vi "xml generate for SFP+_VNA_Full - 副本.vi"(0 "input_array_SDD11_Max":string[](array[string]), 2 "路径":path=path "D:/wmgxml.xml", 3 "input_str_label":string, 4 "input_str_CustomerPN":string, 5 "input_array_SCC11_Max":string[](array[string]), 6 "FilePath":string, 7 "input_array_ILD_Max":string[](array[string]), 8 "FileVer":string, 9 "input_array_TDD11":string[](array[string]), 11 "input_array_TDD22":string[](array[string]), 13 "input_array_time":string[](array[string]), 14 "input_array_impSpec":string[](array[string])) -> ()   [LabVIEW 2011]
panel:
  in  "input_path_dataSource":path
  out "TDD":string
  out "NEXT":string
  out "SCC11":string
  out "SCD21-SDD21":string
  out "ILD":string
  out "SDD11":string
  out "SDD21":string
  in  "RawTXTPath":path
  in  "input_test_results":bool[](array[boolean])
  out "midVar_time":string[](array[string])
  in  "midVar_state":string
  in  "input_str_product":string
  out "midVar_Content":string
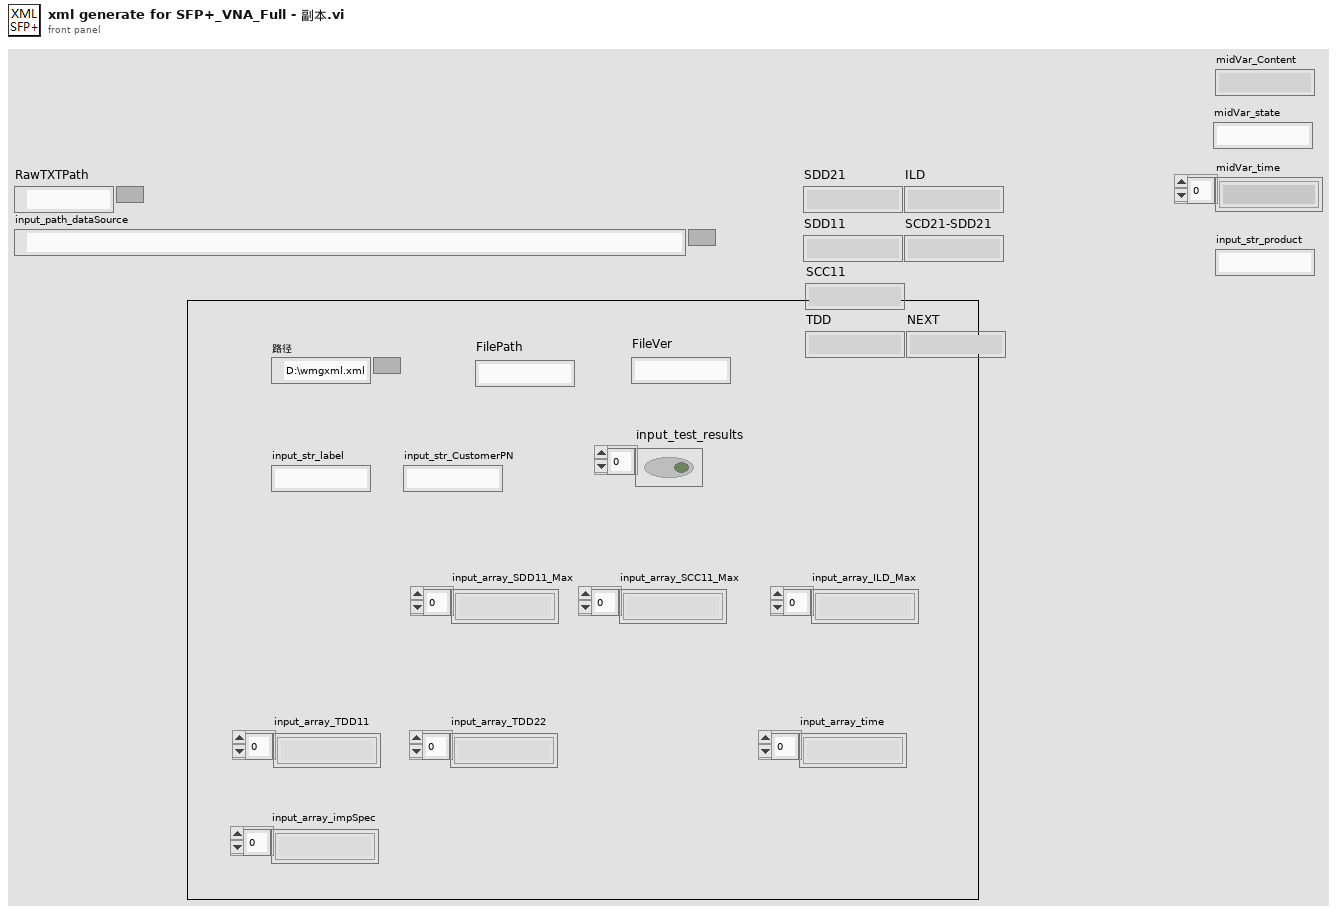
[diagram p1: front panel]
types:
  T1 = enum16{"open", "replace", "create", "open or create", "replace or create", "replace or create with confirmation"}
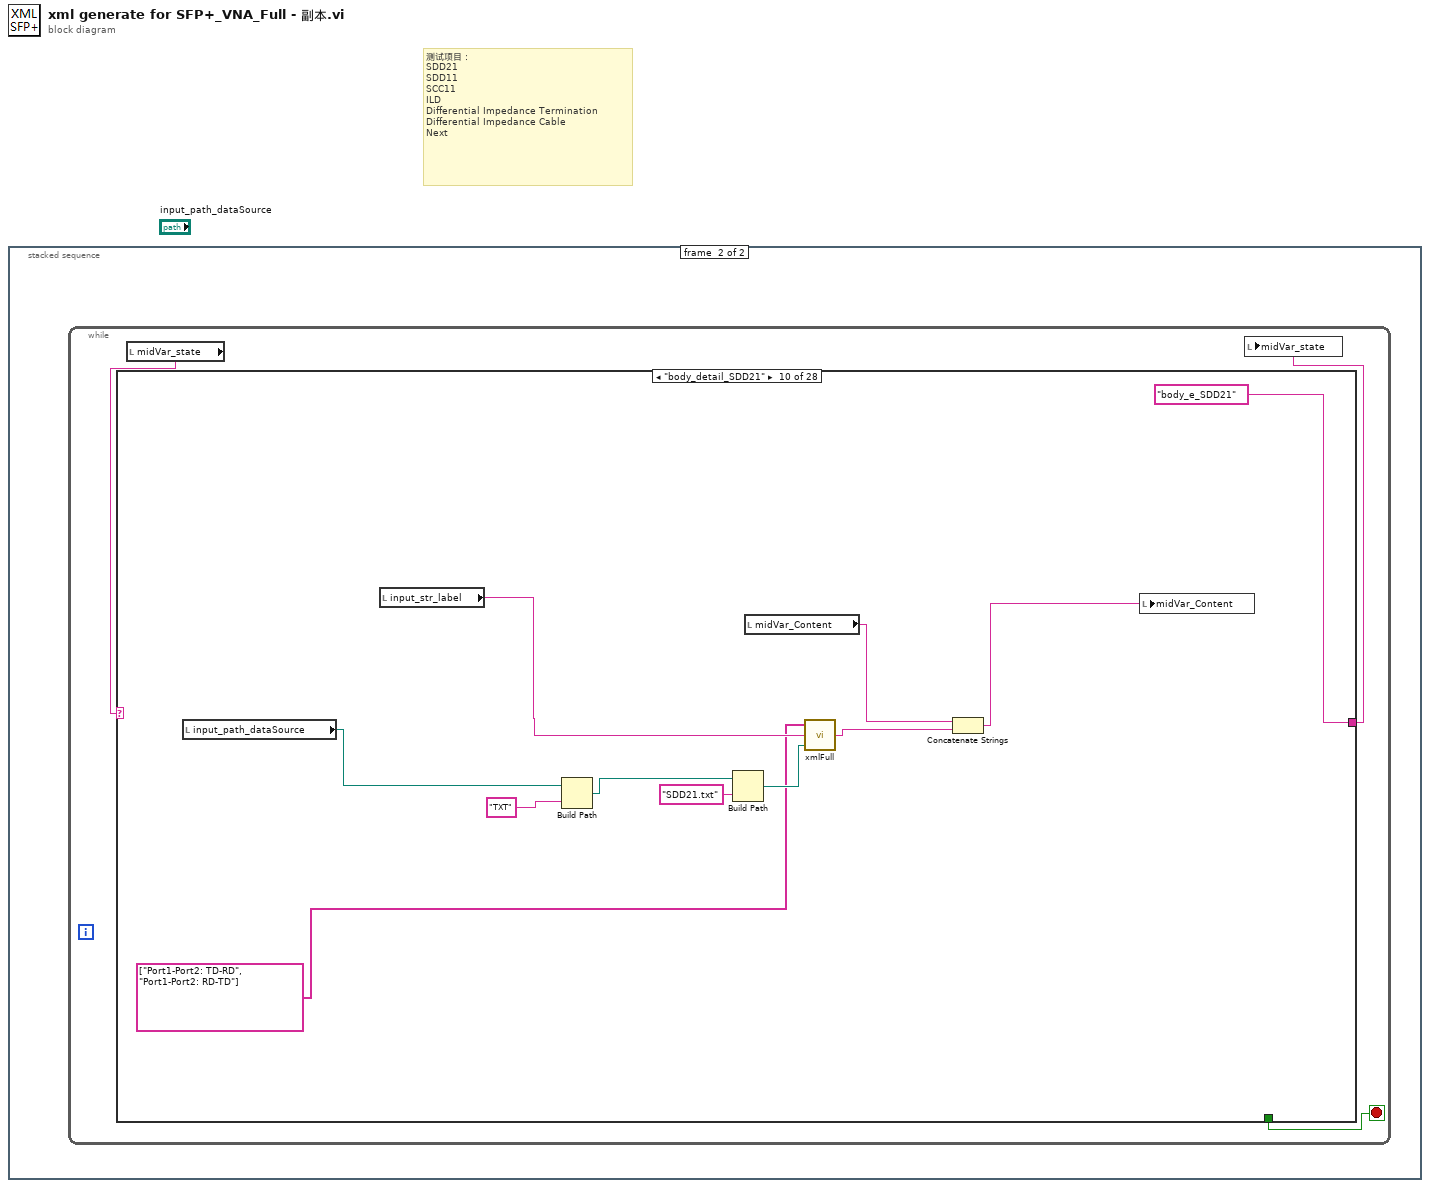
[diagram p0: block diagram]
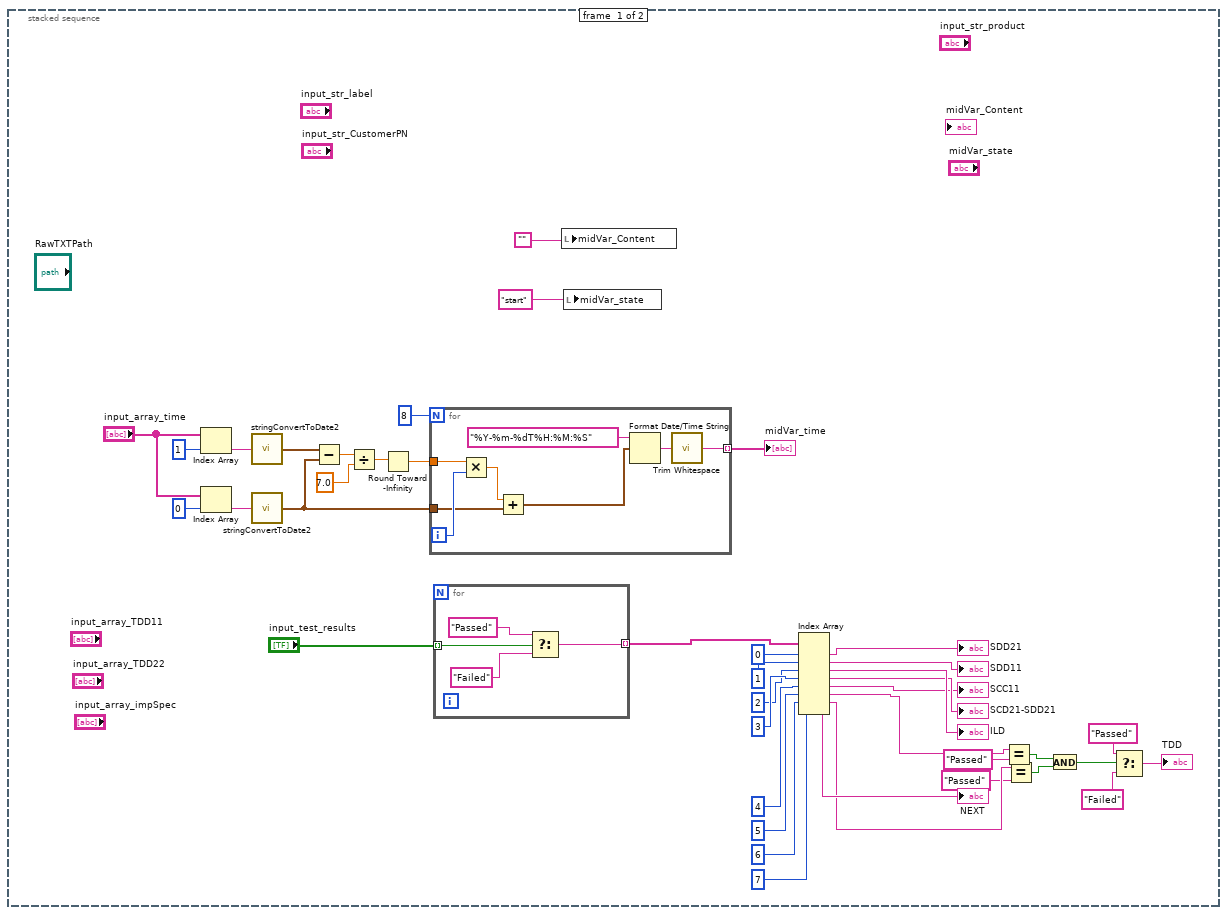
[diagram p2: hidden frame]
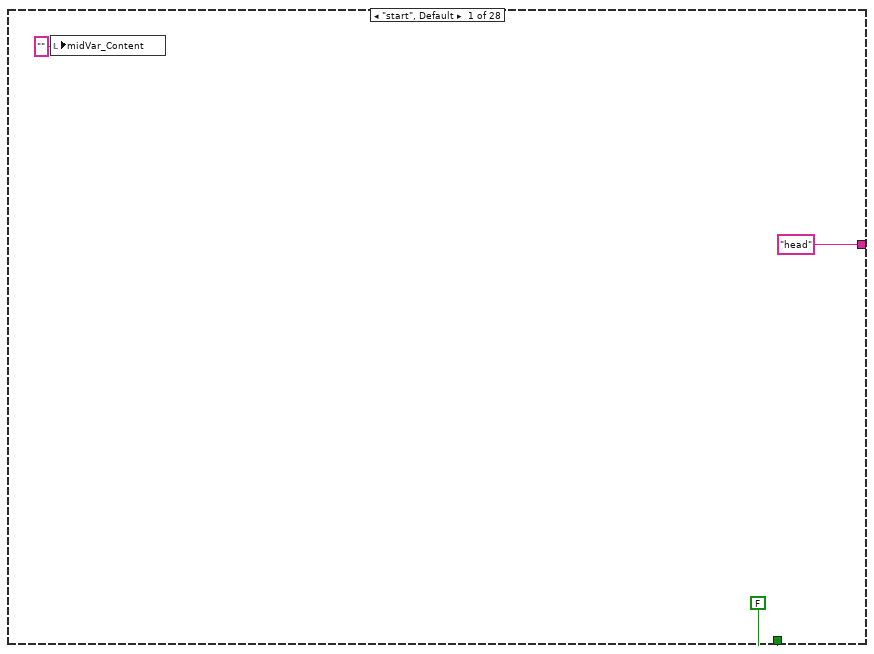
[diagram p3: hidden frame]
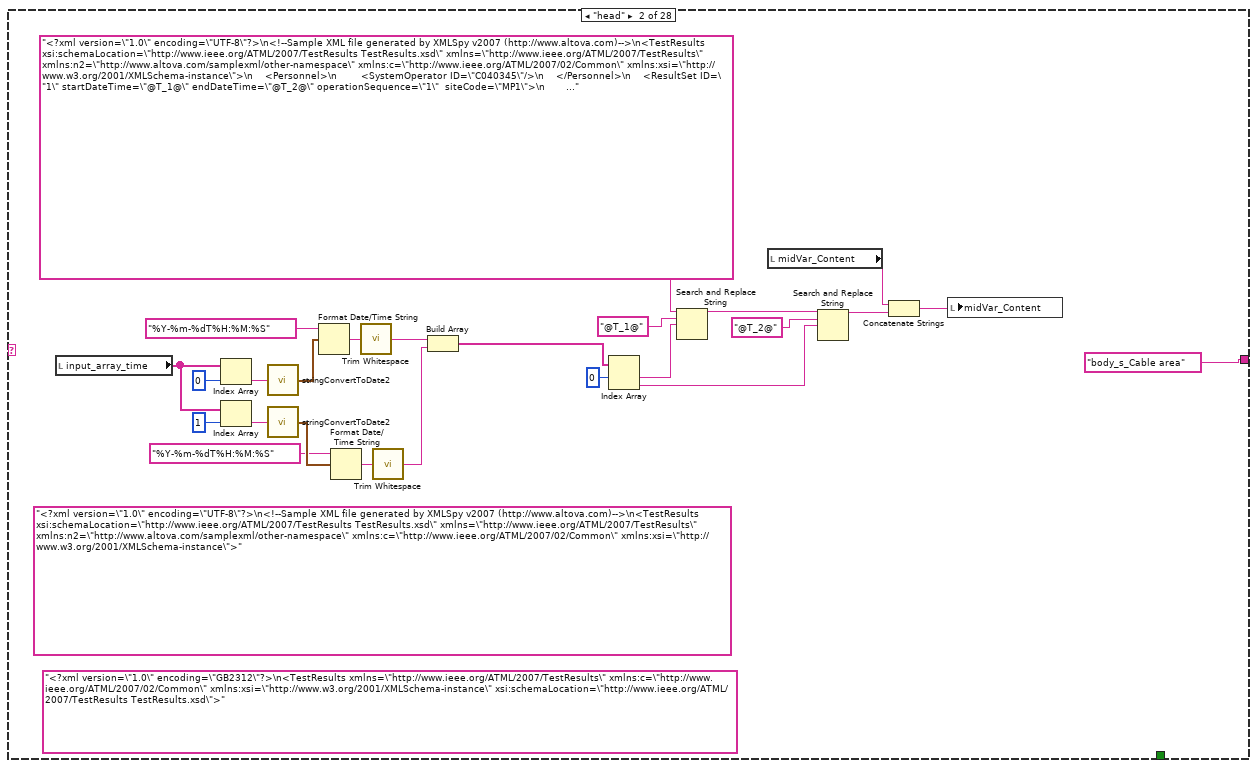
[diagram p4: hidden frame]
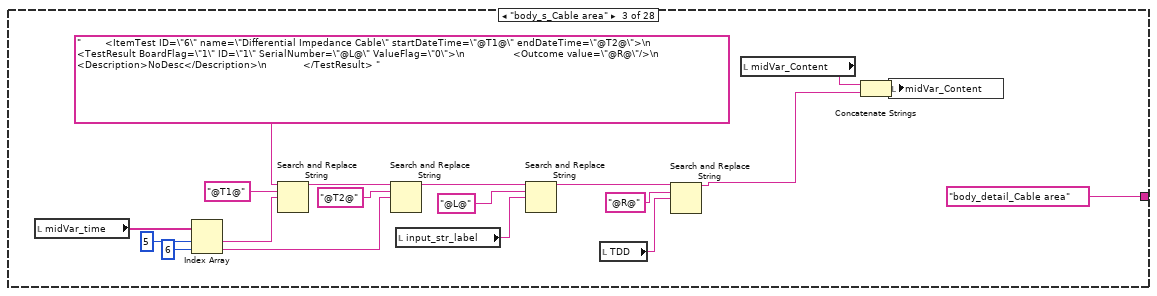
[diagram p5: hidden frame]
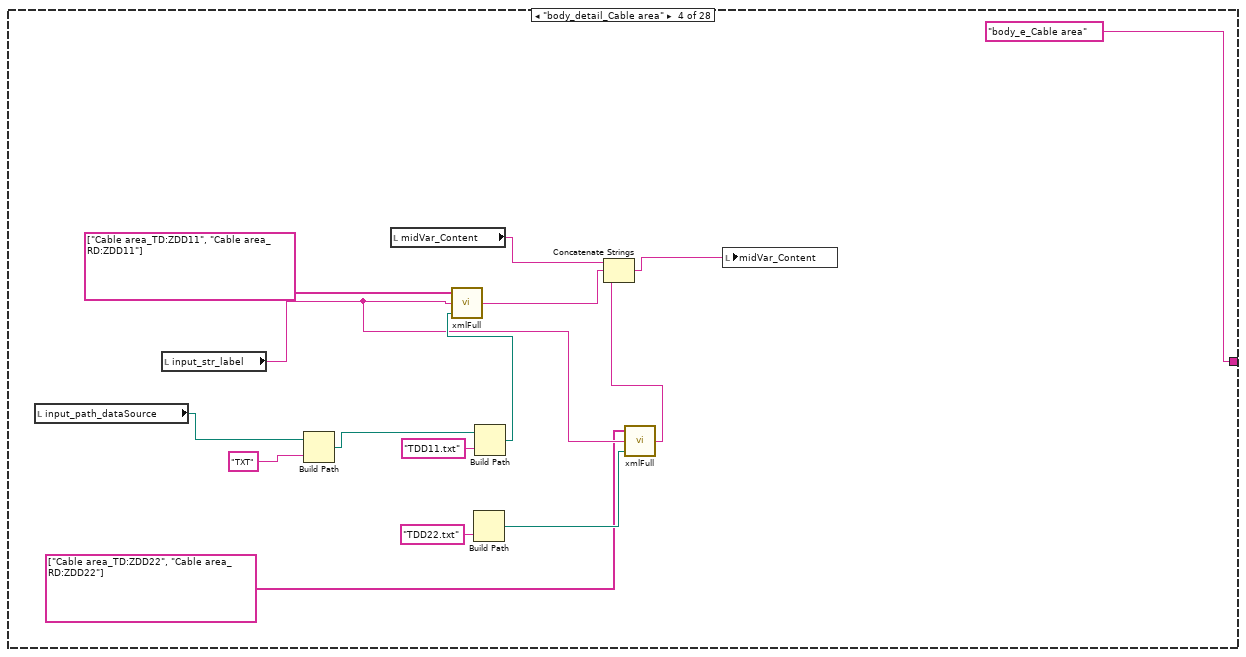
[diagram p6: hidden frame]
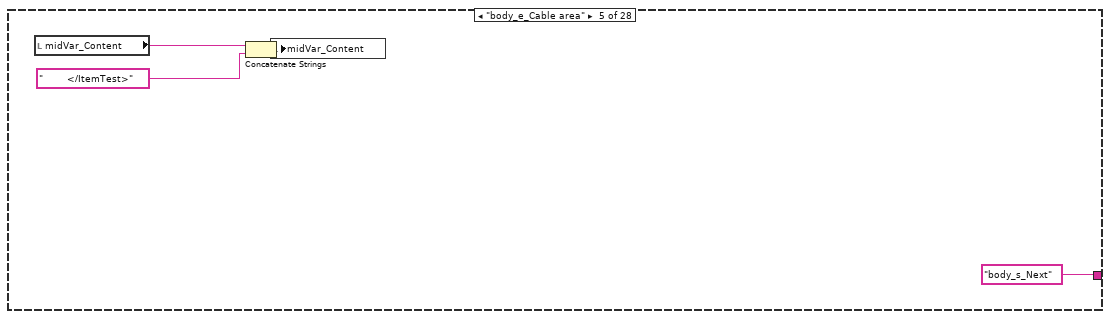
[diagram p7: hidden frame]
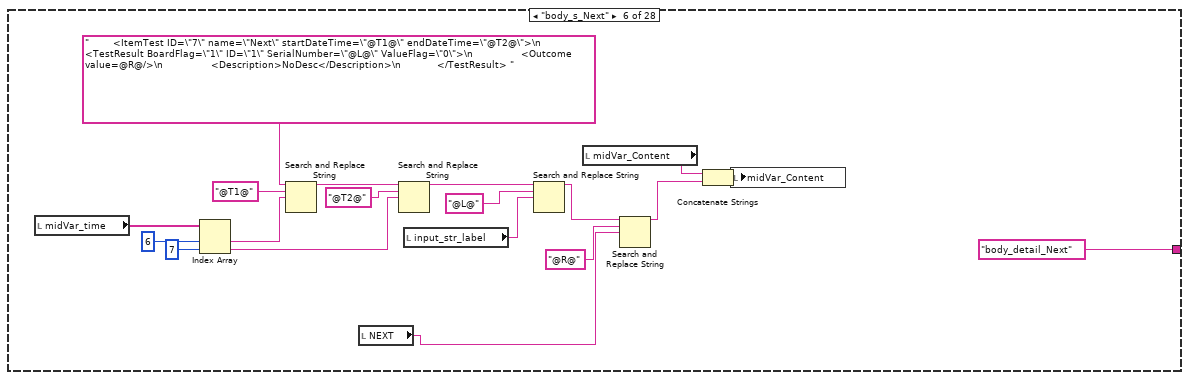
[diagram p8: hidden frame]
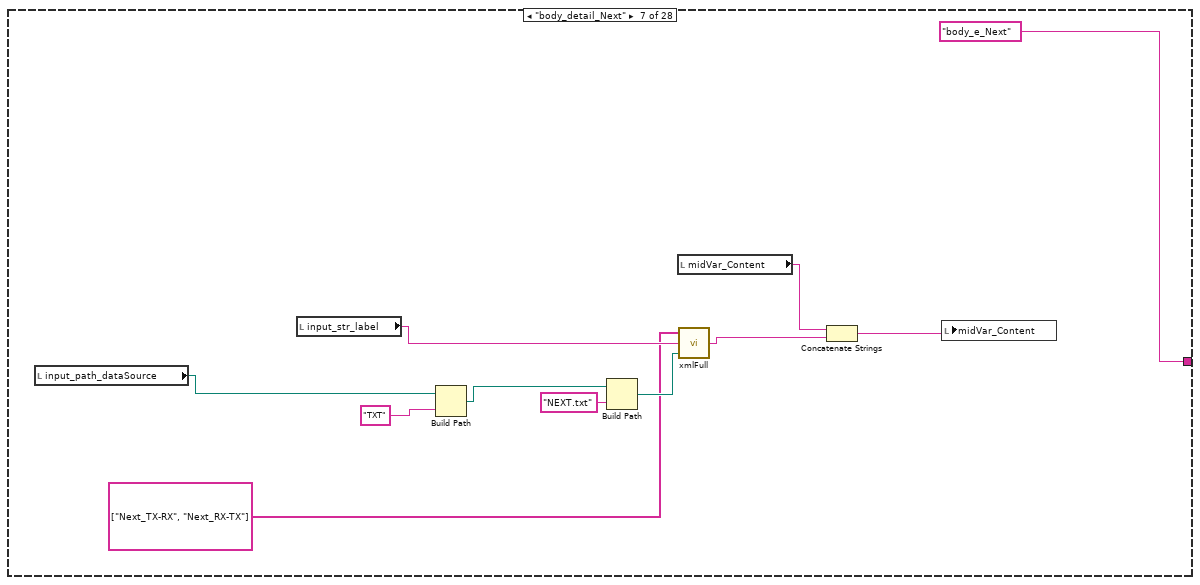
[diagram p9: hidden frame]
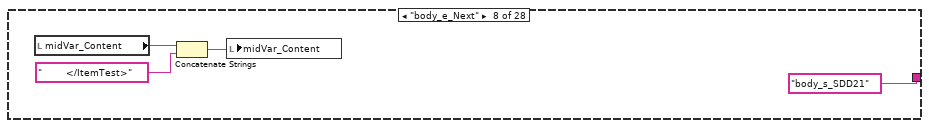
[diagram p10: hidden frame]
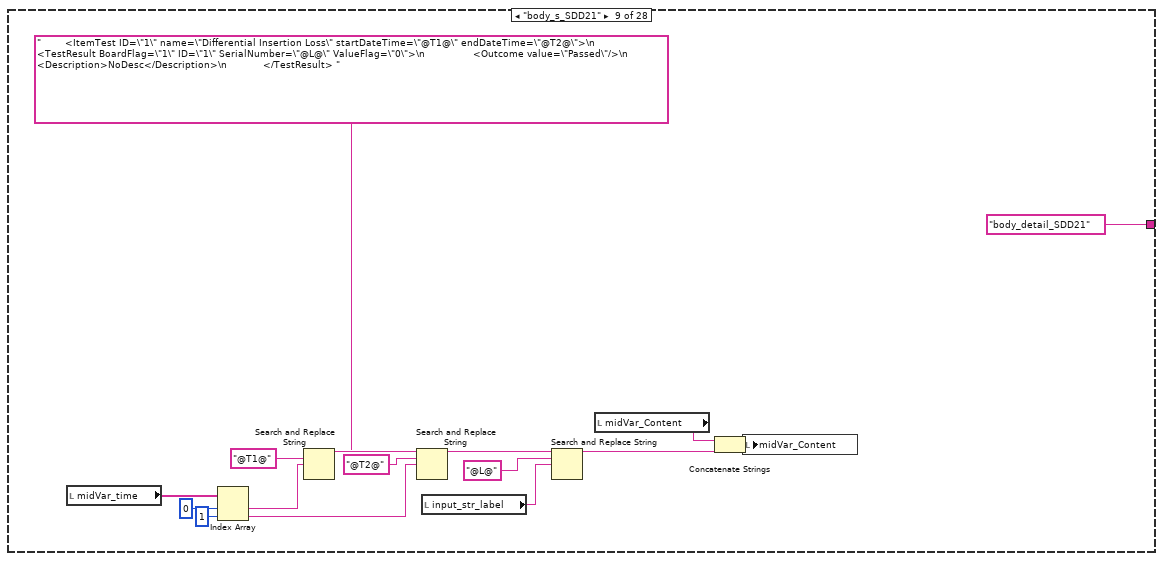
[diagram p11: hidden frame]
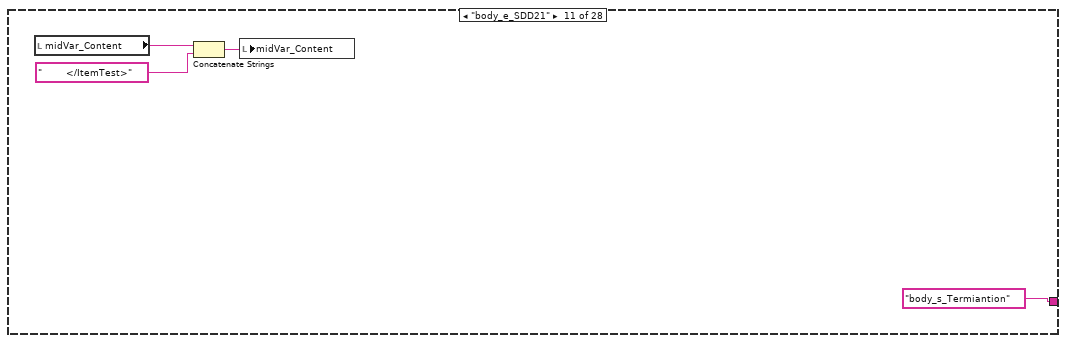
[diagram p12: hidden frame]
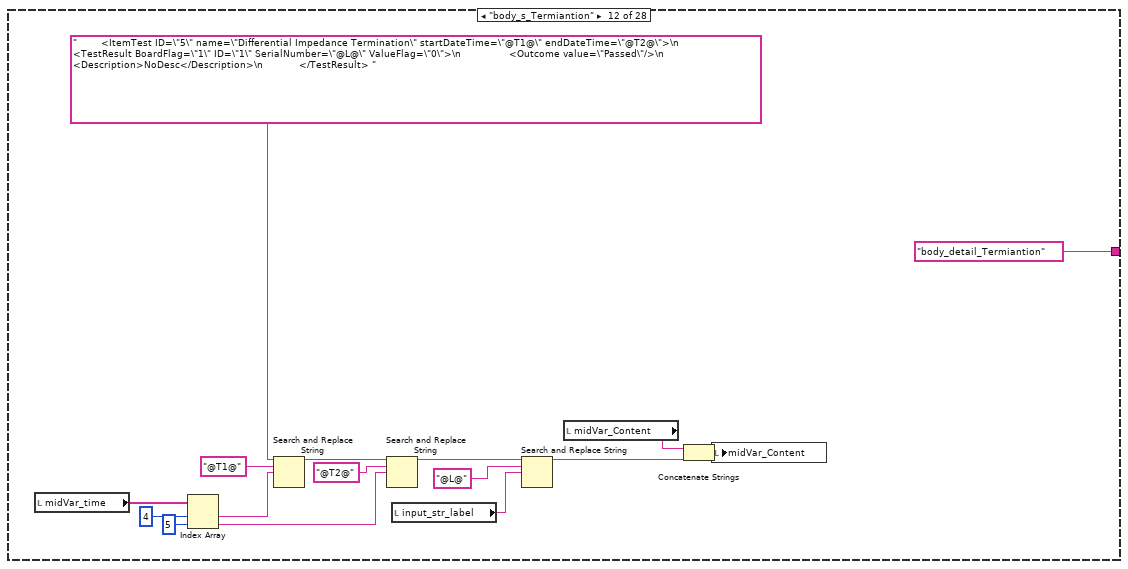
[diagram p13: hidden frame]
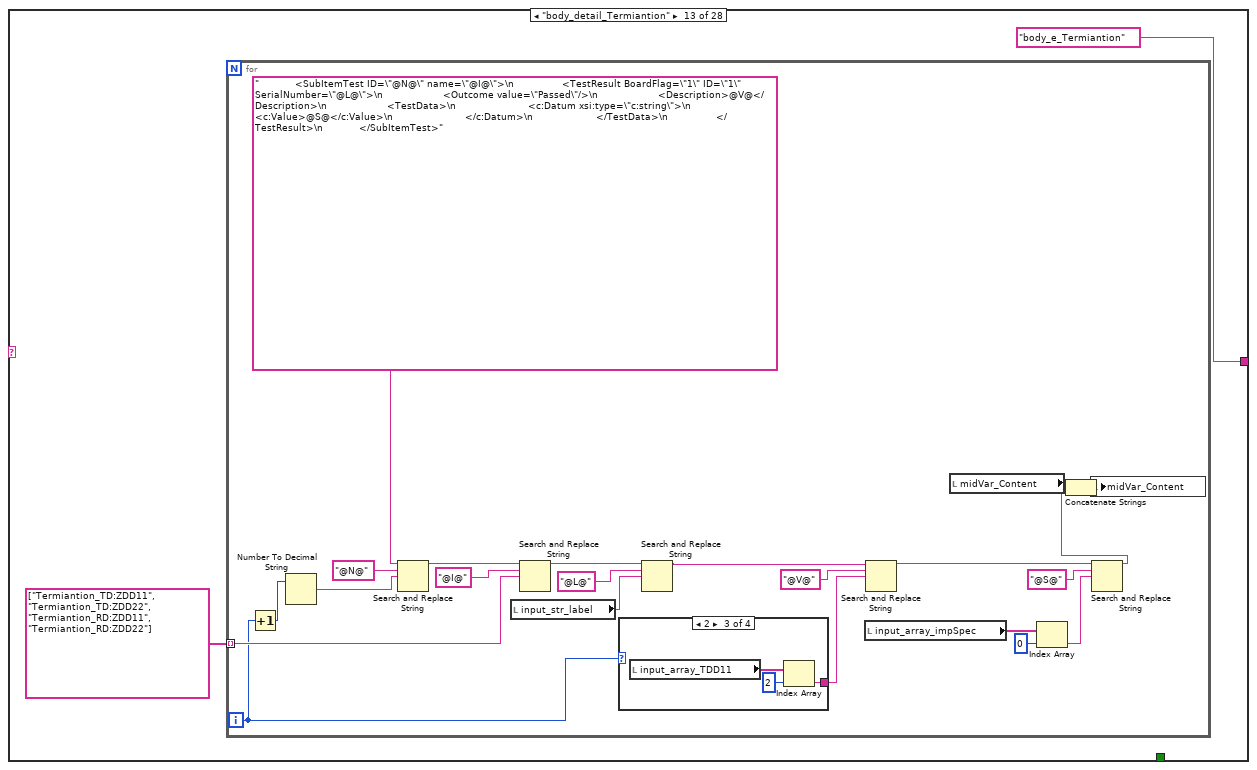
[diagram p14: hidden frame]
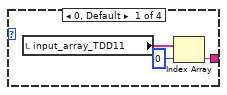
[diagram p15: hidden frame]
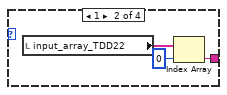
[diagram p16: hidden frame]
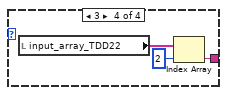
[diagram p17: hidden frame]
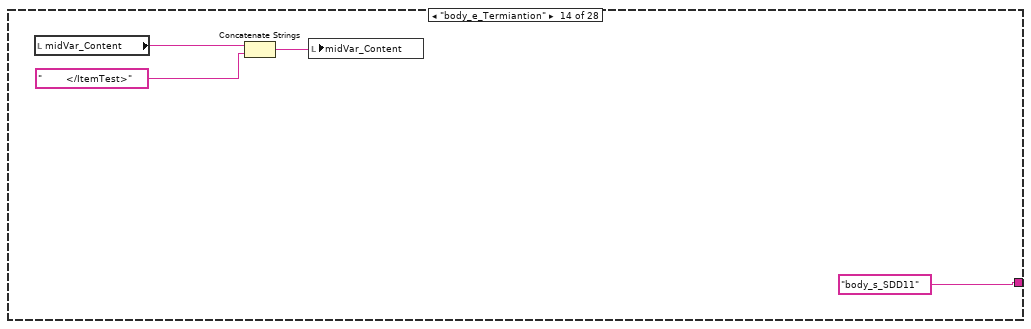
[diagram p18: hidden frame]
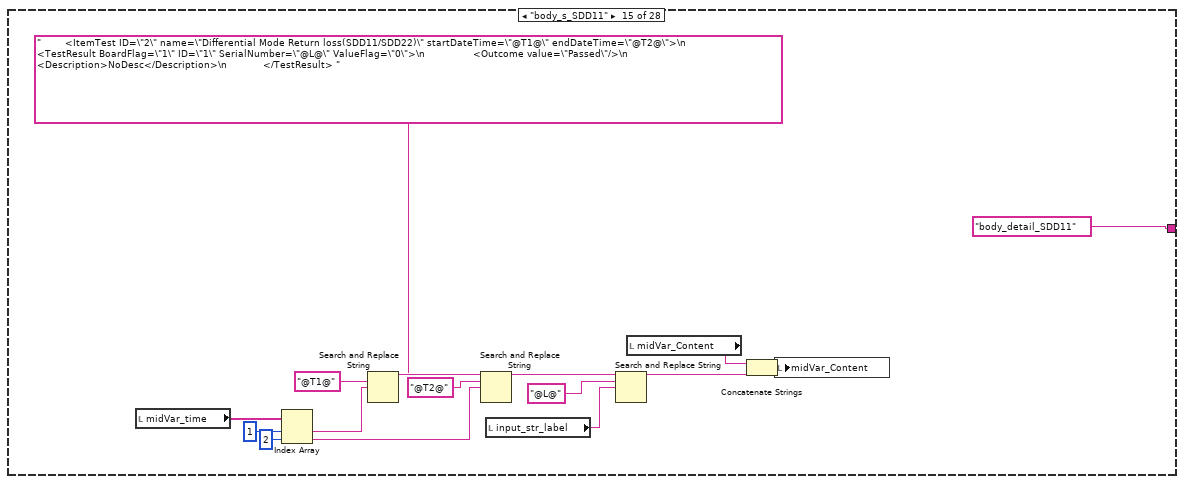
[diagram p19: hidden frame]
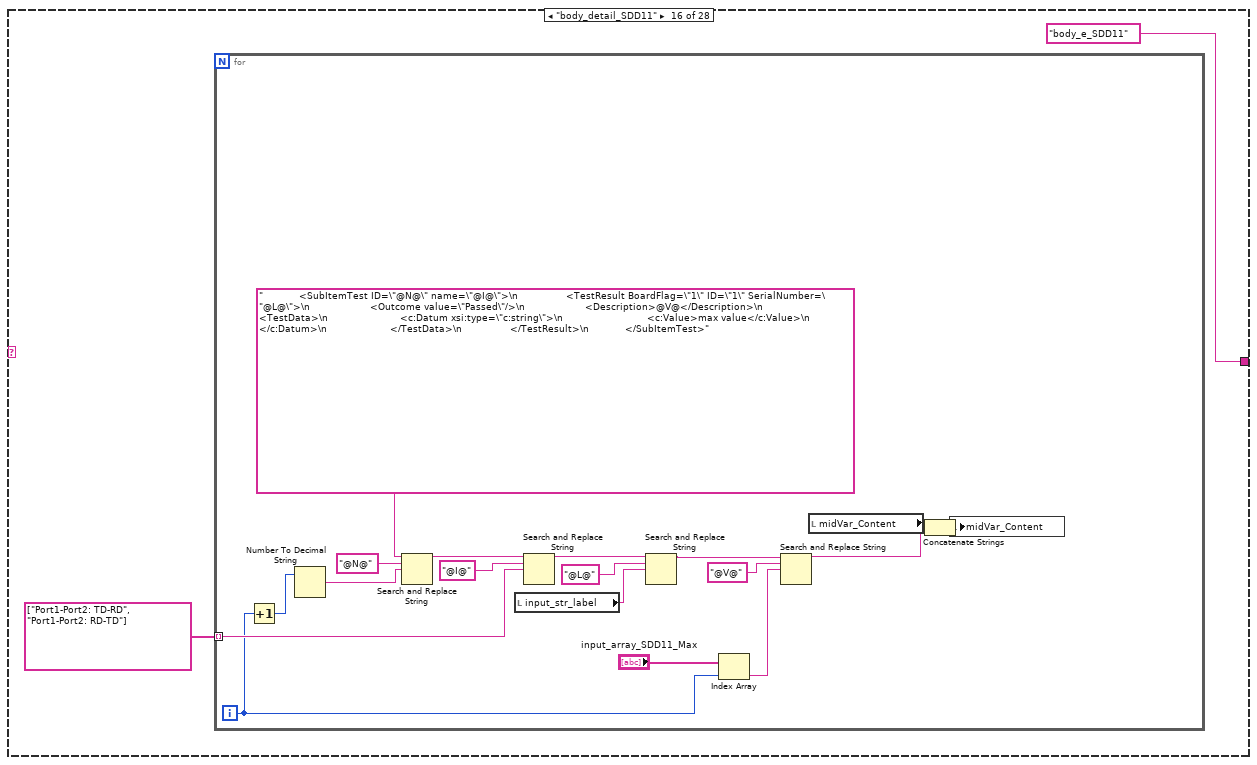
[diagram p20: hidden frame]
diagram:
  # "测试项目：\nSDD21\nSDD11\nSCC11\nILD\nDifferential Impedance Termination\nDifferential Impedance Cable\nNext"
  n1 = stacked-sequence {
    frame #0 {
      n2 = Index Array(array="input_array_time", index=1 ("索引")) -> (element=w30:string)
      n3 = Index Array(array="input_array_time", index=0 ("索引")) -> (element=w31:string)
      n4 = call "stringConvertToDate2.vi"("input_str_yymmdd"=w30) -> ("show_date"=w32:timestamp)
      n5 = call "stringConvertToDate2.vi"("input_str_yymmdd"=w31) -> ("show_date"=w38:timestamp)
      n6 = Subtract(x=w32, y=w38) -> (x-y=w33:dbl)
      n7 = Divide(x=w33, y=7.0) -> (x/y=w35:dbl)
      n8 = Round Toward -Infinity(1:w35) -> (0:w37:dbl)
      n9 = for {
        N: 8 -> [_]
        tunnel: w37 -> [w53]
        tunnel: w38 -> [w51]
        tunnel: [w46] -> w39 mode=indexing
        i -> [w52]
        n10 = Multiply(x=w53, y=w52) -> (x*y=w50:dbl)
        n11 = Add(x=w50, y=w51) -> (x+y=w47:timestamp)
        n12 = Format Date/Time String(time format string (%c)="%Y-%m-%dT%H:%M:%S" ("时间格式字符串(%c)"), seconds (now)=w47) -> (date/time string=w48:string)  [unwired: 1 in]
        n13 = call <vilib>:"Trim Whitespace.vi"("string"=w48) -> ("trimmed string"=w46:string)  [unwired: 1 in]
      }
      "midVar_time" <- w39
      n14 = for {
        tunnel: "input_test_results" -> [w45] mode=indexing
        tunnel: [w42] -> w25 mode=indexing
        n15 = Select(t="Passed", s=w45, f="Failed") -> (s? t:f=w42:string)
      }
      n16 = local write "midVar_Content"("") -> ()
      n17 = local write "midVar_state"("start" ("state")) -> ()
      n18 = Index Array(array=w25, index #1=0 ("索引"), index #2=1 ("索引"), index #3=2 ("索引"), index #4=3 ("索引"), index #5=4 ("索引"), index #6=5 ("索引"), index #7=6 ("索引"), index #8=7 ("索引")) -> (element #1=→"SDD21":string, element #2=→"SDD11":string, element #3=→"ILD":string, element #4=→"SCD21-SDD21":string, element #5=→"SCC11":string, element #6=w10:string, element #7=w8:string, element #8=→"NEXT":string)
      n19 = Equal?(x=w10, y="Passed") -> (x = y?=w6:bool)
      n20 = Equal?(x=w8, y="Passed") -> (x = y?=w5:bool)
      n21 = And(x=w6, y=w5) -> (x .and. y?=w4:bool)
      n22 = Select(t="Passed", s=w4, f="Failed") -> (s? t:f=→"TDD":string)
    }
    frame #1 {
      n23 = while {
        stop <- w54 stop-if-true
        n24 = local read "midVar_state"() -> (w56:string)
        n25 = case shown="\"body_detail_SDD21\"" w56 {
          tunnel: ["head" ("state") "body_s_Cable area" ("state") "body_detail_Cable area" "body_e_Cable area" "body_s_Next" "body_detail_Next" "body_e_Next" "body_s_SDD21" "body_detail_SDD21" "body_e_SDD21" "body_s_Termiantion" "body_detail_Termiantion" "body_e_Termiantion" "body_s_SDD11" "body_detail_SDD11" "body_e_SDD11" "body_s_SCD21-SDD21" "body_detail_SCD21-SDD21" "body_e_SCD21-SDD21" "body_s_ILD" "body_detail_paddle card" ("state") "body_e_SCC11" ("state") _ "body_detail_ILD" "body_e_ILD" "body_s_Termiantion" "end" ("state") "start" ("state")] -> w55
          tunnel: [FALSE _ _ _ _ _ _ _ _ _ _ _ _ _ _ _ _ _ _ _ _ _ _ _ _ _ _ TRUE] -> w54
          frame "start", Default {
            n26 = local write "midVar_Content"("" ("字符串")) -> ()
          }
          frame "head" {
            (unwired) "<?xml version=\"1.0\" encoding=\"GB2312\"?>\n<TestResults xmlns=\"http://www.ieee.org/ATML/2007/TestResults\" xmlns:c=\"http://www.ieee.org/ATML/2007/02/Common\" xmlns:xsi=\"http://www.w3.org/2001/XMLSchema-instance\" xsi:schemaLocation=\"http://www.ieee.org/ATML/2007/TestResults TestResults.xsd\">"
            (unwired) "<?xml version=\"1.0\" encoding=\"UTF-8\"?>\n<!--Sample XML file generated by XMLSpy v2007 (http://www.altova.com)-->\n<TestResults xsi:schemaLocation=\"http://www.ieee.org/ATML/2007/TestResults TestResults.xsd\" xmlns=\"http://www.ieee.org/ATML/2007/TestResults\" xmlns:n2=\"http://www.altova.com/samplexml/other-namespace\" xmlns:c=\"http://www.ieee.org/ATML/2007/02/Common\" xmlns:xsi=\"http://www.w3.org/2001/XMLSchema-instance\">"
            n27 = local read "input_array_time"() -> (w69:string[])
            n28 = Index Array(array=w69, index=0 ("索引")) -> (element=w68:string)
            n29 = Index Array(array=w69, index=1 ("索引")) -> (element=w67:string)
            n30 = call "stringConvertToDate2.vi"("input_str_yymmdd"=w68) -> ("show_date"=w65:timestamp)
            n31 = call "stringConvertToDate2.vi"("input_str_yymmdd"=w67) -> ("show_date"=w64:timestamp)
            n32 = Format Date/Time String(time format string (%c)="%Y-%m-%dT%H:%M:%S" ("时间格式字符串(%c)"), seconds (now)=w65) -> (date/time string=w72:string)  [unwired: 1 in]
            n33 = Format Date/Time String(time format string (%c)="%Y-%m-%dT%H:%M:%S" ("时间格式字符串(%c)"), seconds (now)=w64) -> (date/time string=w66:string)  [unwired: 1 in]
            n34 = call <vilib>:"Trim Whitespace.vi"("string"=w72) -> ("trimmed string"=w62:string)  [unwired: 1 in]
            n35 = call <vilib>:"Trim Whitespace.vi"("string"=w66) -> ("trimmed string"=w61:string)  [unwired: 1 in]
            n36 = Build Array(w62, w61) -> (w60:string[])
            n37 = Index Array(array=w60, index #1=0 ("索引")) -> (element #1=w82:string, element #2=w79:string)  [unwired: 1 in]
            n38 = Search and Replace String(input string="<?xml version=\"1.0\" encoding=\"UTF-8\"?>\n<!--Sample XML file generated by XMLSpy v2007 (http://www.altova.com)-->\n<TestResults xsi:schemaLocation=\"http://www.ieee.org/ATML/2007/TestResults TestResults.xsd\" xmlns=\"http://www.ieee.org/ATML/2007/TestResults\" xmlns:n2=\"http://www.altova.com/samplexml/other-namespace\" xmlns:c=\"http://www.ieee.org/ATML/2007/02/Common\" xmlns:xsi=\"http://www.w3.org/2001/XMLSchema-instance\">\n    <Personnel>\n        <SystemOperator ID=\"C040345\"/>\n    </Personnel>\n    <ResultSet ID=\"1\" startDateTime=\"@T_1@\" endDateTime=\"@T_2@\" operationSequence=\"1\"  siteCode=\"MP1\">\n        <Description>CMZ00A2R</Description>\n        <TestResult BoardFlag=\"1\" ID=\"1\">\n            <Outcome value=\"Passed\"/>\n        </TestResult>", search string="@T_1@" ("搜索字符串"), replace string=w82) -> (result string=w81:string)  [unwired: 5 in, 3 out]
            n39 = local read "midVar_Content"() -> (w77:string)
            n40 = Search and Replace String(input string=w81, search string="@T_2@" ("搜索字符串"), replace string=w79) -> (result string=w74:string)  [unwired: 5 in, 3 out]
            n41 = Concatenate Strings(w77, w74) -> (w76:string)
            n42 = local write "midVar_Content"(w76) -> ()
          }
          frame "body_s_Cable area" {
            n43 = local read "midVar_time"() -> (w90:string[])
            n44 = Index Array(array=w90, index #1=5 ("索引"), index #2=6 ("索引")) -> (element #1=w101:string, element #2=w98:string)
            n45 = Search and Replace String(input string="        <ItemTest ID=\"6\" name=\"Differential Impedance Cable\" startDateTime=\"@T1@\" endDateTime=\"@T2@\">\n            <TestResult BoardFlag=\"1\" ID=\"1\" SerialNumber=\"@L@\" ValueFlag=\"0\">\n                <Outcome value=\"@R@\"/>\n                <Description>NoDesc</Description>\n            </TestResult> ", search string="@T1@" ("搜索字符串"), replace string=w101) -> (result string=w100:string)  [unwired: 5 in, 3 out]
            n46 = Search and Replace String(input string=w100, search string="@T2@" ("搜索字符串"), replace string=w98) -> (result string=w93:string)  [unwired: 5 in, 3 out]
            n47 = local read "input_str_label"() -> (w92:string)
            n48 = Search and Replace String(input string=w93, search string="@L@" ("搜索字符串"), replace string=w92) -> (result string=w88:string)  [unwired: 5 in, 3 out]
            n49 = local read "TDD"() -> (w85:string)
            n50 = Search and Replace String(input string=w88, search string="@R@" ("搜索字符串"), replace string=w85) -> (result string=w87:string)  [unwired: 5 in, 3 out]
            n51 = local read "midVar_Content"() -> (w97:string)
            n52 = Concatenate Strings(w97, w87) -> (w96:string)
            n53 = local write "midVar_Content"(w96) -> ()
          }
          frame "body_detail_Cable area" {
            n54 = local read "input_path_dataSource"() -> (w104:path)
            n55 = local read "input_str_label"() -> (w107:string)
            n56 = Build Path(base path=w104, name or relative path="TXT" ("名称或相对路径")) -> (appended path=w112:path)
            n57 = local read "midVar_Content"() -> (w117:string)
            n58 = Build Path(name or relative path="TDD22.txt" ("名称或相对路径")) -> (appended path=w108:path)  [unwired: 1 in]
            n59 = Build Path(base path=w112, name or relative path="TDD11.txt" ("名称或相对路径")) -> (appended path=w110:path)
            n60 = call "xmlFull.vi"("file path (dialog if empty)"=w110, "SN"=w107, "数组"=string[] ["Cable area_TD:ZDD11", "Cable area_RD:ZDD11"]) -> ("OutPutXml"=w115:string)
            n61 = call "xmlFull.vi"("file path (dialog if empty)"=w108, "SN"=w107, "数组"=string[] ["Cable area_TD:ZDD22", "Cable area_RD:ZDD22"]) -> ("OutPutXml"=w105:string)
            n62 = Concatenate Strings(w117, w115, w105) -> (w116:string)
            n63 = local write "midVar_Content"(w116) -> ()
          }
          frame "body_e_Cable area" {
            n64 = local read "midVar_Content"() -> (w122:string)
            n65 = Concatenate Strings(w122, "        </ItemTest>") -> (w121:string)
            n66 = local write "midVar_Content"(w121) -> ()
          }
          frame "body_s_Next" {
            n67 = local read "midVar_time"() -> (w128:string[])
            n68 = Index Array(array=w128, index #1=6 ("索引"), index #2=7 ("索引")) -> (element #1=w139:string, element #2=w136:string)
            n69 = Search and Replace String(input string="        <ItemTest ID=\"7\" name=\"Next\" startDateTime=\"@T1@\" endDateTime=\"@T2@\">\n            <TestResult BoardFlag=\"1\" ID=\"1\" SerialNumber=\"@L@\" ValueFlag=\"0\">\n                <Outcome value=@R@/>\n                <Description>NoDesc</Description>\n            </TestResult> ", search string="@T1@" ("搜索字符串"), replace string=w139) -> (result string=w138:string)  [unwired: 5 in, 3 out]
            n70 = local read "NEXT"() -> (w126:string)
            n71 = Search and Replace String(input string=w138, search string="@T2@" ("搜索字符串"), replace string=w136) -> (result string=w131:string)  [unwired: 5 in, 3 out]
            n72 = local read "input_str_label"() -> (w130:string)
            n73 = Search and Replace String(input string=w131, search string="@L@" ("搜索字符串"), replace string=w130) -> (result string=w124:string)  [unwired: 5 in, 3 out]
            n74 = local read "midVar_Content"() -> (w135:string)
            n75 = Search and Replace String(input string=w124, search string="@R@" ("搜索字符串"), replace string=w126) -> (result string=w123:string)  [unwired: 5 in, 3 out]
            n76 = Concatenate Strings(w135, w123) -> (w134:string)
            n77 = local write "midVar_Content"(w134) -> ()
          }
          frame "body_detail_Next" {
            n78 = local read "input_path_dataSource"() -> (w148:path)
            n79 = local read "input_str_label"() -> (w146:string)
            n80 = Build Path(base path=w148, name or relative path="TXT" ("名称或相对路径")) -> (appended path=w150:path)
            n81 = Build Path(base path=w150, name or relative path="NEXT.txt" ("名称或相对路径")) -> (appended path=w147:path)
            n82 = local read "midVar_Content"() -> (w143:string)
            n83 = call "xmlFull.vi"("file path (dialog if empty)"=w147, "SN"=w146, "数组"=string[] ["Next_TX-RX", "Next_RX-TX"]) -> ("OutPutXml"=w144:string)
            n84 = Concatenate Strings(w143, w144) -> (w142:string)
            n85 = local write "midVar_Content"(w142) -> ()
          }
          frame "body_e_Next" {
            n86 = local read "midVar_Content"() -> (w156:string)
            n87 = Concatenate Strings(w156, "        </ItemTest>") -> (w155:string)
            n88 = local write "midVar_Content"(w155) -> ()
          }
          frame "body_s_SDD21" {
            n89 = local read "midVar_time"() -> (w158:string[])
            n90 = Index Array(array=w158, index #1=0 ("索引"), index #2=1 ("索引")) -> (element #1=w170:string, element #2=w167:string)
            n91 = Search and Replace String(input string="        <ItemTest ID=\"1\" name=\"Differential Insertion Loss\" startDateTime=\"@T1@\" endDateTime=\"@T2@\">\n            <TestResult BoardFlag=\"1\" ID=\"1\" SerialNumber=\"@L@\" ValueFlag=\"0\">\n                <Outcome value=\"Passed\"/>\n                <Description>NoDesc</Description>\n            </TestResult> ", search string="@T1@" ("搜索字符串"), replace string=w170) -> (result string=w169:string)  [unwired: 5 in, 3 out]
            n92 = Search and Replace String(input string=w169, search string="@T2@" ("搜索字符串"), replace string=w167) -> (result string=w162:string)  [unwired: 5 in, 3 out]
            n93 = local read "input_str_label"() -> (w161:string)
            n94 = Search and Replace String(input string=w162, search string="@L@" ("搜索字符串"), replace string=w161) -> (result string=w159:string)  [unwired: 5 in, 3 out]
            n95 = local read "midVar_Content"() -> (w166:string)
            n96 = Concatenate Strings(w166, w159) -> (w165:string)
            n97 = local write "midVar_Content"(w165) -> ()
          }
          frame "body_detail_SDD21" {
            n98 = local read "input_path_dataSource"() -> (w177:path)
            n99 = local read "input_str_label"() -> (w176:string)
            n100 = Build Path(base path=w177, name or relative path="TXT" ("名称或相对路径")) -> (appended path=w181:path)
            n101 = Build Path(base path=w181, name or relative path="SDD21.txt" ("名称或相对路径")) -> (appended path=w179:path)
            n102 = local read "midVar_Content"() -> (w174:string)
            n103 = call "xmlFull.vi"("file path (dialog if empty)"=w179, "SN"=w176, "数组"=string[] ["Port1-Port2: TD-RD", "Port1-Port2: RD-TD"]) -> ("OutPutXml"=w178:string)
            n104 = Concatenate Strings(w174, w178) -> (w175:string)
            n105 = local write "midVar_Content"(w175) -> ()
          }
          frame "body_e_SDD21" {
            n106 = local read "midVar_Content"() -> (w187:string)
            n107 = Concatenate Strings(w187, "        </ItemTest>") -> (w186:string)
            n108 = local write "midVar_Content"(w186) -> ()
          }
          frame "body_s_Termiantion" {
            n109 = local read "midVar_time"() -> (w189:string[])
            n110 = Index Array(array=w189, index #1=4 ("索引"), index #2=5 ("索引")) -> (element #1=w201:string, element #2=w198:string)
            n111 = Search and Replace String(input string="        <ItemTest ID=\"5\" name=\"Differential Impedance Termination\" startDateTime=\"@T1@\" endDateTime=\"@T2@\">\n            <TestResult BoardFlag=\"1\" ID=\"1\" SerialNumber=\"@L@\" ValueFlag=\"0\">\n                <Outcome value=\"Passed\"/>\n                <Description>NoDesc</Description>\n            </TestResult> ", search string="@T1@" ("搜索字符串"), replace string=w201) -> (result string=w200:string)  [unwired: 5 in, 3 out]
            n112 = Search and Replace String(input string=w200, search string="@T2@" ("搜索字符串"), replace string=w198) -> (result string=w193:string)  [unwired: 5 in, 3 out]
            n113 = local read "input_str_label"() -> (w192:string)
            n114 = Search and Replace String(input string=w193, search string="@L@" ("搜索字符串"), replace string=w192) -> (result string=w190:string)  [unwired: 5 in, 3 out]
            n115 = local read "midVar_Content"() -> (w197:string)
            n116 = Concatenate Strings(w197, w190) -> (w196:string)
            n117 = local write "midVar_Content"(w196) -> ()
          }
          frame "body_detail_Termiantion" {
            n118 = for {
              tunnel: string[] ["Termiantion_TD:ZDD11", "Termiantion_TD:ZDD22", "Termiantion_RD:ZDD11", "Termiantion_RD:ZDD22"] -> [w222] mode=indexing
              i -> [w209]
              n119 = Increment(x=w209) -> (x+1=w211:i32)
              n120 = Number To Decimal String(number=w211) -> (decimal integer string=w225:string)  [unwired: 1 in]
              n121 = Search and Replace String(input string="            <SubItemTest ID=\"@N@\" name=\"@I@\">\n                <TestResult BoardFlag=\"1\" ID=\"1\" SerialNumber=\"@L@\">\n                    <Outcome value=\"Passed\"/>\n                    <Description>@V@</Description>\n                    <TestData>\n                        <c:Datum xsi:type=\"c:string\">\n                            <c:Value>@S@</c:Value>\n                        </c:Datum>\n                     </TestData>\n                </TestResult>\n            </SubItemTest>", search string="@N@" ("搜索字符串"), replace string=w225) -> (result string=w224:string)  [unwired: 5 in, 3 out]
              n122 = local read "input_str_label"() -> (w219:string)
              n123 = Search and Replace String(input string=w224, search string="@I@" ("搜索字符串"), replace string=w222) -> (result string=w221:string)  [unwired: 5 in, 3 out]
              n124 = case shown="2" w209 {
                tunnel: [w230 w233 w236 w239] -> w216
                frame 0, Default {
                  n125 = local read "input_array_TDD11"() -> (w229:string[])
                  n126 = Index Array(array=w229, index=0 ("索引")) -> (element=w230:string)
                }
                frame 1 {
                  n127 = local read "input_array_TDD22"() -> (w232:string[])
                  n128 = Index Array(array=w232, index=0 ("索引")) -> (element=w233:string)
                }
                frame 2 {
                  n129 = local read "input_array_TDD11"() -> (w235:string[])
                  n130 = Index Array(array=w235, index=2 ("索引")) -> (element=w236:string)
                }
                frame 3 {
                  n131 = local read "input_array_TDD22"() -> (w238:string[])
                  n132 = Index Array(array=w238, index=2 ("索引")) -> (element=w239:string)
                }
              }
              n133 = Search and Replace String(input string=w221, search string="@L@" ("搜索字符串"), replace string=w219) -> (result string=w210:string)  [unwired: 5 in, 3 out]
              n134 = local read "input_array_impSpec"() -> (w207:string[])
              n135 = Search and Replace String(input string=w210, search string="@V@" ("搜索字符串"), replace string=w216) -> (result string=w208:string)  [unwired: 5 in, 3 out]
              n136 = local read "midVar_Content"() -> (w218:string)
              n137 = Index Array(array=w207, index=0 ("索引")) -> (element=w206:string)
              n138 = Search and Replace String(input string=w208, search string="@S@" ("搜索字符串"), replace string=w206) -> (result string=w213:string)  [unwired: 5 in, 3 out]
              n139 = Concatenate Strings(w218, w213) -> (w212:string)
              n140 = local write "midVar_Content"(w212) -> ()
            }
          }
          frame "body_e_Termiantion" {
            n141 = local read "midVar_Content"() -> (w243:string)
            n142 = Concatenate Strings(w243, "        </ItemTest>") -> (w242:string)
            n143 = local write "midVar_Content"(w242) -> ()
          }
          frame "body_s_SDD11" {
            n144 = local read "midVar_time"() -> (w245:string[])
            n145 = Index Array(array=w245, index #1=1 ("索引"), index #2=2 ("索引")) -> (element #1=w257:string, element #2=w254:string)
            n146 = Search and Replace String(input string="        <ItemTest ID=\"2\" name=\"Differential Mode Return loss(SDD11/SDD22)\" startDateTime=\"@T1@\" endDateTime=\"@T2@\">\n            <TestResult BoardFlag=\"1\" ID=\"1\" SerialNumber=\"@L@\" ValueFlag=\"0\">\n                <Outcome value=\"Passed\"/>\n                <Description>NoDesc</Description>\n            </TestResult> ", search string="@T1@" ("搜索字符串"), replace string=w257) -> (result string=w256:string)  [unwired: 5 in, 3 out]
            n147 = Search and Replace String(input string=w256, search string="@T2@" ("搜索字符串"), replace string=w254) -> (result string=w249:string)  [unwired: 5 in, 3 out]
            n148 = local read "input_str_label"() -> (w248:string)
            n149 = Search and Replace String(input string=w249, search string="@L@" ("搜索字符串"), replace string=w248) -> (result string=w246:string)  [unwired: 5 in, 3 out]
            n150 = local read "midVar_Content"() -> (w253:string)
            n151 = Concatenate Strings(w253, w246) -> (w252:string)
            n152 = local write "midVar_Content"(w252) -> ()
          }
          frame "body_detail_SDD11" {
            n153 = for {
              tunnel: string[] ["Port1-Port2: TD-RD", "Port1-Port2: RD-TD"] -> [w274] mode=indexing
              i -> [w264]
              n154 = Increment(x=w264) -> (x+1=w266:i32)
              n155 = Number To Decimal String(number=w266) -> (decimal integer string=w277:string)  [unwired: 1 in]
              n156 = Search and Replace String(input string="            <SubItemTest ID=\"@N@\" name=\"@I@\">\n                <TestResult BoardFlag=\"1\" ID=\"1\" SerialNumber=\"@L@\">\n                    <Outcome value=\"Passed\"/>\n                    <Description>@V@</Description>\n                    <TestData>\n                        <c:Datum xsi:type=\"c:string\">\n                            <c:Value>max value</c:Value>\n                        </c:Datum>\n                     </TestData>\n                </TestResult>\n            </SubItemTest>", search string="@N@" ("搜索字符串"), replace string=w277) -> (result string=w276:string)  [unwired: 5 in, 3 out]
              n157 = local read "input_str_label"() -> (w271:string)
              n158 = Search and Replace String(input string=w276, search string="@I@" ("搜索字符串"), replace string=w274) -> (result string=w273:string)  [unwired: 5 in, 3 out]
              n159 = Search and Replace String(input string=w273, search string="@L@" ("搜索字符串"), replace string=w271) -> (result string=w265:string)  [unwired: 5 in, 3 out]
              n160 = Index Array(array="input_array_SDD11_Max", index=w264) -> (element=w268:string)
              n161 = Search and Replace String(input string=w265, search string="@V@" ("搜索字符串"), replace string=w268) -> (result string=w262:string)  [unwired: 5 in, 3 out]
              n162 = local read "midVar_Content"() -> (w270:string)
              n163 = Concatenate Strings(w270, w262) -> (w267:string)
              n164 = local write "midVar_Content"(w267) -> ()
            }
          }
          frame "body_e_SDD11" {
            n165 = local read "midVar_Content"() -> (w283:string)
            n166 = Concatenate Strings(w283, "        </ItemTest>") -> (w282:string)
            n167 = local write "midVar_Content"(w282) -> ()
          }
          frame "body_s_SCD21-SDD21" {
            n168 = local read "midVar_time"() -> (w285:string[])
            n169 = Index Array(array=w285, index #1=2 ("索引"), index #2=3 ("索引")) -> (element #1=w297:string, element #2=w294:string)
            n170 = Search and Replace String(input string="        <ItemTest ID=\"3\" name=\"Jitter From (SCD21-SDD21)\" startDateTime=\"@T1@\" endDateTime=\"@T2@\">\n            <TestResult BoardFlag=\"1\" ID=\"1\" SerialNumber=\"@L@\" ValueFlag=\"0\">\n                <Outcome value=\"Passed\"/>\n                <Description>NoDesc</Description>\n            </TestResult> ", search string="@T1@" ("搜索字符串"), replace string=w297) -> (result string=w296:string)  [unwired: 5 in, 3 out]
            n171 = Search and Replace String(input string=w296, search string="@T2@" ("搜索字符串"), replace string=w294) -> (result string=w289:string)  [unwired: 5 in, 3 out]
            n172 = local read "input_str_label"() -> (w288:string)
            n173 = Search and Replace String(input string=w289, search string="@L@" ("搜索字符串"), replace string=w288) -> (result string=w286:string)  [unwired: 5 in, 3 out]
            n174 = local read "midVar_Content"() -> (w293:string)
            n175 = Concatenate Strings(w293, w286) -> (w292:string)
            n176 = local write "midVar_Content"(w292) -> ()
          }
          frame "body_detail_SCD21-SDD21" {
            n177 = for {
              tunnel: string[] ["Port1-Port2: TD-RD", "Port1-Port2: RD-TD"] -> [w315] mode=indexing
              i -> [w302]
              n178 = Increment(x=w302) -> (x+1=w307:i32)
              n179 = Number To Decimal String(number=w307) -> (decimal integer string=w318:string)  [unwired: 1 in]
              n180 = Search and Replace String(input string="            <SubItemTest ID=\"@N@\" name=\"@I@\">\n                <TestResult BoardFlag=\"1\" ID=\"1\" SerialNumber=\"@L@\">\n                    <Outcome value=\"Passed\"/>\n                    <Description>@V@</Description>\n                    <TestData>\n                        <c:Datum xsi:type=\"c:string\">\n                            <c:Value>max value</c:Value>\n                        </c:Datum>\n                     </TestData>\n                </TestResult>\n            </SubItemTest>", search string="@N@" ("搜索字符串"), replace string=w318) -> (result string=w317:string)  [unwired: 5 in, 3 out]
              n181 = local read "input_str_label"() -> (w312:string)
              n182 = Search and Replace String(input string=w317, search string="@I@" ("搜索字符串"), replace string=w315) -> (result string=w314:string)  [unwired: 5 in, 3 out]
              n183 = Search and Replace String(input string=w314, search string="@L@" ("搜索字符串"), replace string=w312) -> (result string=w305:string)  [unwired: 5 in, 3 out]
              n184 = Index Array(array="input_array_SCC11_Max", index=w302) -> (element=w309:string)
              n185 = local read "midVar_Content"() -> (w311:string)
              n186 = Search and Replace String(input string=w305, search string="@V@" ("搜索字符串"), replace string=w309) -> (result string=w304:string)  [unwired: 5 in, 3 out]
              n187 = Concatenate Strings(w311, w304) -> (w308:string)
              n188 = local write "midVar_Content"(w308) -> ()
            }
          }
          frame "body_e_SCD21-SDD21" {
            n189 = local read "midVar_Content"() -> (w323:string)
            n190 = Concatenate Strings(w323, "        </ItemTest>") -> (w322:string)
            n191 = local write "midVar_Content"(w322) -> ()
          }
          frame "body_s_paddle card" {
          }
          frame "body_detail_paddle card" {
          }
          frame "body_e_paddle card" {
          }
          frame "body_s_ILD" {
            n192 = local read "midVar_time"() -> (w327:string[])
            n193 = Index Array(array=w327, index #1=3 ("索引"), index #2=4 ("索引")) -> (element #1=w339:string, element #2=w336:string)
            n194 = Search and Replace String(input string="        <ItemTest ID=\"4\" name=\"Insertion Loss Deviation\" startDateTime=\"@T1@\" endDateTime=\"@T2@\">\n            <TestResult BoardFlag=\"1\" ID=\"1\" SerialNumber=\"@L@\" ValueFlag=\"0\">\n                <Outcome value=\"Passed\"/>\n                <Description>NoDesc</Description>\n            </TestResult> ", search string="@T1@" ("搜索字符串"), replace string=w339) -> (result string=w338:string)  [unwired: 5 in, 3 out]
            n195 = Search and Replace String(input string=w338, search string="@T2@" ("搜索字符串"), replace string=w336) -> (result string=w331:string)  [unwired: 5 in, 3 out]
            n196 = local read "input_str_label"() -> (w330:string)
            n197 = Search and Replace String(input string=w331, search string="@L@" ("搜索字符串"), replace string=w330) -> (result string=w328:string)  [unwired: 5 in, 3 out]
            n198 = local read "midVar_Content"() -> (w335:string)
            n199 = Concatenate Strings(w335, w328) -> (w334:string)
            n200 = local write "midVar_Content"(w334) -> ()
          }
          frame "body_detail_ILD" {
            n201 = for {
              tunnel: string[] ["Port1-Port2: TD-RD", "Port1-Port2: RD-TD"] -> [w357] mode=indexing
              i -> [w345]
              n202 = Increment(x=w345) -> (x+1=w349:i32)
              n203 = Number To Decimal String(number=w349) -> (decimal integer string=w360:string)  [unwired: 1 in]
              n204 = Search and Replace String(input string="            <SubItemTest ID=\"@N@\" name=\"@I@\">\n                <TestResult BoardFlag=\"1\" ID=\"1\" SerialNumber=\"@L@\">\n                    <Outcome value=\"Passed\"/>\n                    <Description>@V@</Description>\n                    <TestData>\n                        <c:Datum xsi:type=\"c:string\">\n                            <c:Value>max value</c:Value>\n                        </c:Datum>\n                     </TestData>\n                </TestResult>\n            </SubItemTest>", search string="@N@" ("搜索字符串"), replace string=w360) -> (result string=w359:string)  [unwired: 5 in, 3 out]
              n205 = local read "input_str_label"() -> (w354:string)
              n206 = Search and Replace String(input string=w359, search string="@I@" ("搜索字符串"), replace string=w357) -> (result string=w356:string)  [unwired: 5 in, 3 out]
              n207 = Search and Replace String(input string=w356, search string="@L@" ("搜索字符串"), replace string=w354) -> (result string=w347:string)  [unwired: 5 in, 3 out]
              n208 = Index Array(array="input_array_ILD_Max", index=w345) -> (element=w351:string)
              n209 = Search and Replace String(input string=w347, search string="@V@" ("搜索字符串"), replace string=w351) -> (result string=w344:string)  [unwired: 5 in, 3 out]
              n210 = local read "midVar_Content"() -> (w353:string)
              n211 = Concatenate Strings(w353, w344) -> (w350:string)
              n212 = local write "midVar_Content"(w350) -> ()
            }
          }
          frame "body_e_ILD" {
            n213 = local read "midVar_Content"() -> (w365:string)
            n214 = Concatenate Strings(w365, "        </ItemTest>") -> (w364:string)
            n215 = local write "midVar_Content"(w364) -> ()
          }
          frame "tail" {
            # "</ResultSet>\n    <TestProgram Productline=\"XT-113\" Product=\"SFP+\">\n        <c:Definition name=\"HPTS\" version=\"6.0\">\n            <c:Description>NoDesc</c:Description> \n        </c:Definition>\n    </TestProgram>\n    <!--  ATE--> \n    <TestStation AteName=\"TDR\" AteVersion=\"1.001\" /> \n    <!--  SerialNumber--> \n    <UUT UutType=\"hardware\">\n        <SerialNumber>@L@</SerialNumber> \n        <ItemName>SFP+</ItemName>\n        <ItemCode>@C@</ItemCode> \n    </UUT>\n    <WorkOrder>\n        <WorkItem name=\"a\">\n            <c:Datum xsi:type=\"c:string\">\n                <c:Value>SPZS06311C1</c:Value> \n            </c:Datum>\n        </WorkItem>\n    </WorkOrder>\n</TestResults"
            n216 = Concatenate Strings("\"" ("字符串"), "FileVer", "\"" ("字符串")) -> (w370:string)
            n217 = local read "input_str_product"() -> (w392:string)
            n218 = Search and Replace String(input string="    </ResultSet>\n    <TestProgram Productline=\"XT-113\" Product=\"SFP+\">\n        <c:Definition name=\"VNA\" version=@Ver@>\n            <c:Description>@Path@</c:Description> \n        </c:Definition>\n    </TestProgram>\n    <!--  ATE--> \n    <TestStation AteName=@PCName@ AteVersion=\"1.001\" /> \n    <!--  SerialNumber--> \n    <UUT UutType=\"hardware\">\n        <SerialNumber>@L@</SerialNumber> \n        <ItemName>SFP+</ItemName>\n        <ItemCode>@C@</ItemCode> \n    </UUT>\n    <WorkOrder>\n        <WorkItem name=\"a\">\n            <c:Datum xsi:type=\"c:string\">\n                <c:Value>SPZS06311C1</c:Value> \n            </c:Datum>\n        </WorkItem>\n    </WorkOrder>\n</TestResults>", search string="@Ver@" ("搜索字符串"), replace string=w370) -> (result string=w379:string)  [unwired: 5 in, 3 out]
            n219 = call "PCsName.vi"() -> ("Computer Name"=w369:string)
            n220 = Search and Replace String(input string=w379, search string="@Path@" ("搜索字符串"), replace string="FilePath") -> (result string=w377:string)  [unwired: 5 in, 3 out]
            n221 = local read "input_str_label"() -> (w389:string)
            n222 = Concatenate Strings("\"" ("字符串"), w369, "\"" ("字符串")) -> (w366:string)
            n223 = Search and Replace String(input string=w377, search string="@PCName@" ("搜索字符串"), replace string=w366) -> (result string=w375:string)  [unwired: 5 in, 3 out]
            n224 = Search and Replace String(input string=w375, search string="@P@" ("搜索字符串"), replace string=w392) -> (result string=w391:string)  [unwired: 5 in, 3 out]
            n225 = Search and Replace String(input string=w391, search string="@L@" ("搜索字符串"), replace string=w389) -> (result string=w384:string)  [unwired: 5 in, 3 out]
            n226 = local read "input_str_CustomerPN"() -> (w382:string)
            n227 = local read "midVar_Content"() -> (w388:string)
            n228 = Search and Replace String(input string=w384, search string="@C@" ("搜索字符串"), replace string=w382) -> (result string=w385:string)  [unwired: 5 in, 3 out]
            n229 = Concatenate Strings(w388, w385) -> (w387:string)
            n230 = local write "midVar_Content"(w387) -> ()
          }
          frame "end" {
            n231 = local read "midVar_Content"() -> (w396:string)
            n232 = Open/Create/Replace File(file path (use dialog)="路径", operation (0:open)=T1."open or create" ("操作(0:open)")) -> (refnum out=w398:refnum<file>)  [unwired: 4 in, 2 out]
            n233 = Write to Text File(file (use dialog)=w398, text=w396) -> (refnum out=w397:refnum<file>)  [unwired: 2 in, 2 out]
            n234 = Close File(refnum=w397) -> ()  [unwired: 1 in, 2 out]
          }
        }
        n235 = local write "midVar_state"(w55) -> ()
      }
    }
  }
